vi "Queue Receive.vi"(11 "Hello World Queue in":refnum<class "Hello World Queue.lvclass">) -> (2 "Msg Strategy":refnum<class "Msg Strategy.lvclass">, 3 "Hello World Queue out":refnum<class "Hello World Queue.lvclass">)   [LabVIEW 2021, in "Hello World Queue.lvlib" / "Hello World Queue.lvclass"]
uses:
  Hello World Queue.lvclass
  jettl/Msg Strategy/Msg Strategy.lvclass
  Hello World Queue.lvclass/Hello World Queue.ctl
  jettl/jettl/Queue jettl/Queue jettl.lvclass
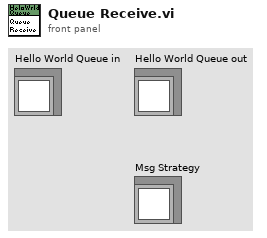
[diagram p1: front panel]
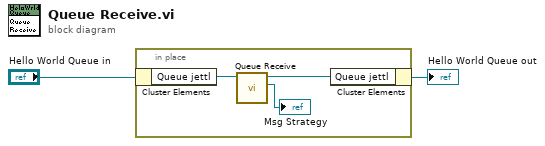
[diagram p0: block diagram]
diagram:
  n1 = in-place {
    n2 = in-place-cluster #1("Hello World Queue in") -> ("Queue jettl"=w5:refnum<class "Queue jettl.lvclass">)
    n3 = call-dynamic "Queue Receive.vi"("Queue jettl in"=w5) -> ("Msg Strategy"=→"Msg Strategy":refnum<class "Msg Strategy.lvclass">, "Queue jettl out"=w4:refnum<class "Queue jettl.lvclass">)  [unwired: 9 in]
    n4 = in-place-cluster #1("Queue jettl"=w4) -> (→"Hello World Queue out":refnum<class "Hello World Queue.lvclass">)
  }
